vi "加载控件.vi"(8 "error in (no error)":errorcluster caption="错误输入（无错误）", 11 "程序 输入":refnum<class "程序.lvclass">) -> (0 "error out":errorcluster caption="错误输出", 3 "程序 输出":refnum<class "程序.lvclass">)   [LabVIEW 2018, in "程序.lvclass"]
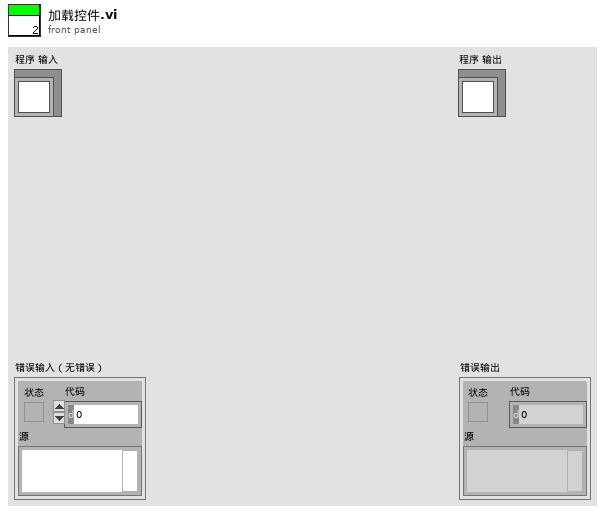
[diagram p1: front panel]
types:
  T1 = typedef "imagedata.ctl" = cluster{"image type":i32, "image depth":i32, "image":u8[], "mask":u8[], "colors":u32[], "Rectangle":cluster{"left":i16, "top":i16, "right":i16, "bottom":i16}}
  T2 = cluster{"new picture":picture, string, string, string}
  T3 = cluster{"new picture":picture, string, string, string}[]
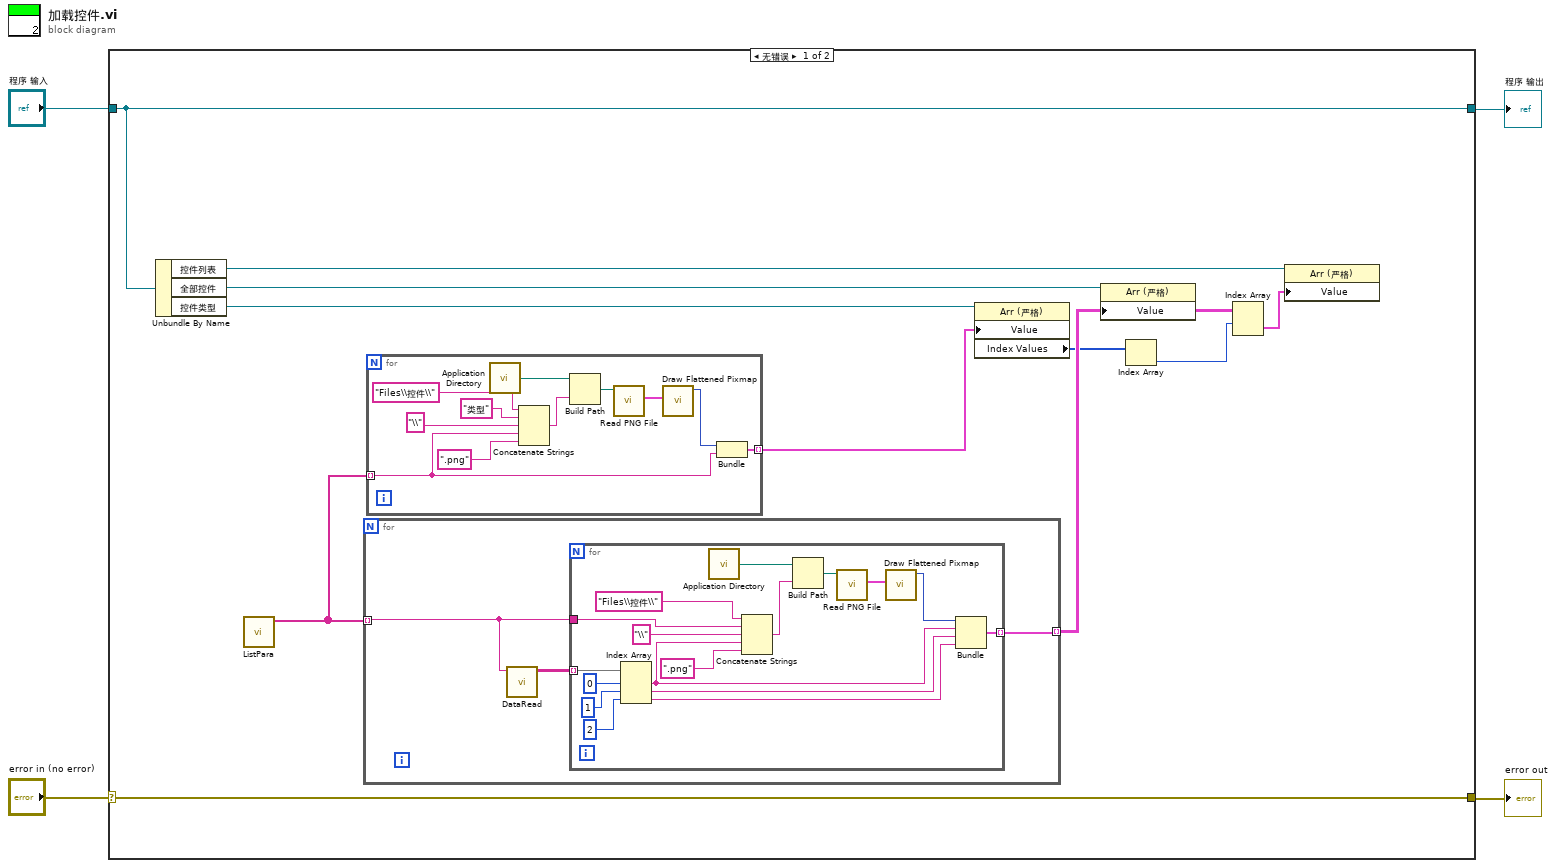
[diagram p0: block diagram]
diagram:
  n1 = case shown="无错误" "error in (no error)" {
    selector: "error in (no error)" -> [w15 w48]
    tunnel: [w15 w48] -> w3
    tunnel: [w14 w47] -> w1
    tunnel: "程序 输入" -> [w14 w47]
    frame No Error {
      n2 = Unbundle By Name(w14) -> ("控件列表"=w9:refnum<vi>, "全部控件"=w13:refnum<vi>, "控件类型"=w11:refnum<vi>)
      n3 = call "ListPara.vi"() -> ("Paras"=w12:string[])  [unwired: 11 in]
      n4 = for {
        tunnel: w12 -> [w27] mode=indexing
        tunnel: [w28] -> w8 mode=indexing
        n5 = call "DataRead.vi"("段名"=w27) -> ("数据"=w29:string[][])  [unwired: 10 in]
        n6 = for {
          tunnel: w29 -> [w38] mode=indexing
          tunnel: [w39] -> w28 mode=indexing
          tunnel: w27 -> [w30]
          n7 = Index Array(array=w38, index #1=0 ("索引"), index #2=1 ("索引"), index #3=2 ("索引")) -> (element #1=w37:string, element #2=w34:string, element #3=w32:string)
          n8 = call <vilib>:"Application Directory.vi"() -> ("Application Directory"=w46:path)
          n9 = Concatenate Strings("Files\\控件\\" ("名称或相对路径"), w30, "\\" ("字符串"), w37, ".png" ("字符串")) -> (w44:string)
          n10 = Build Path(base path=w46, name or relative path=w44) -> (appended path=w42:path)
          n11 = call <vilib>:"Read PNG File.vi"("path to PNG file"=w42) -> ("image data"=w41:T1)  [unwired: 8 in, 2 out]
          n12 = call <vilib>:"Draw Flattened Pixmap.vi"("image data"=w41) -> ("new picture"=w40:picture)  [unwired: 8 in]
          n13 = Bundle("new picture"=w40, w37, w34, w32) -> (w39:T2)  [unwired: 1 in]
        }
      }
      n14 = for {
        tunnel: w12 -> [w17] mode=indexing
        tunnel: [w16] -> w10 mode=indexing
        n15 = call <vilib>:"Application Directory.vi"() -> ("Application Directory"=w20:path)
        n16 = Concatenate Strings("Files\\控件\\" ("名称或相对路径"), "类型" ("字符串"), "\\" ("字符串"), w17, ".png" ("字符串")) -> (w22:string)
        n17 = Build Path(base path=w20, name or relative path=w22) -> (appended path=w24:path)
        n18 = call <vilib>:"Read PNG File.vi"("path to PNG file"=w24) -> ("image data"=w25:T1)  [unwired: 8 in, 2 out]
        n19 = call <vilib>:"Draw Flattened Pixmap.vi"("image data"=w25) -> ("new picture"=w18:picture)  [unwired: 8 in]
        n20 = Bundle("new picture"=w18, "String"=w17) -> (w16:cluster{"new picture":picture, "String":string})  [unwired: 1 in]
      }
      n21 = property class="Arr (严格)"(reference=w11, "Value"=w10) -> ("Index Values"=w6:u32[])  [unwired: 1 in, 2 out]
      n22 = property class="Arr (严格)"(reference=w13, "Value"=w8) -> ()  [unwired: 1 in, 2 out]
      n23 = Index Array(array=w6) -> (element=w5:u32)  [unwired: 1 in]
      n24 = Index Array(array=w8, index (row)=w5) -> (element=w7:T3)  [unwired: 1 in]
      n25 = property class="Arr (严格)"(reference=w9, "Value"=w7) -> ()  [unwired: 1 in, 2 out]
    }
    frame Error {
    }
  }
  "error out" <- w3
  "程序 输出" <- w1
